vi "Set Snake Direction.vi"(8 "error in (no error)":errorcluster, 10 "Direction":T1, 11 "Snake in":refnum<class "Snake.lvclass">) -> (0 "error out":errorcluster, 3 "Snake out":refnum<class "Snake.lvclass">)   [LabVIEW 2018, in "Snake.lvclass"]
uses:
  Snake.lvclass
  Type Defs/Direction.ctl
  Snake.lvclass/Snake.ctl
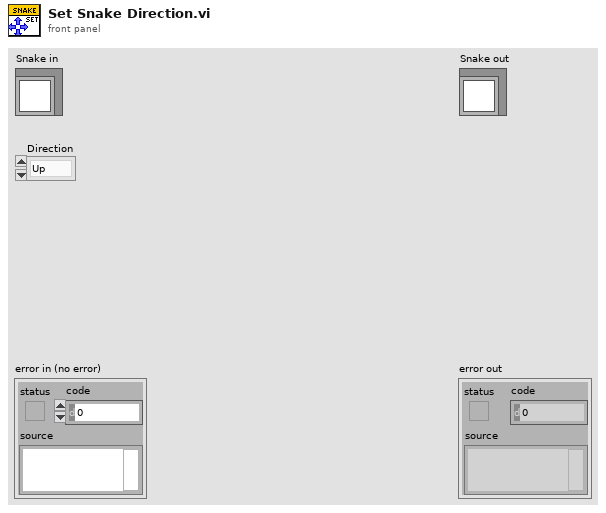
[diagram p1: front panel]
types:
  T1 = typedef "Direction.ctl" = enum16{"Up", "Down", "Left", "Right"}
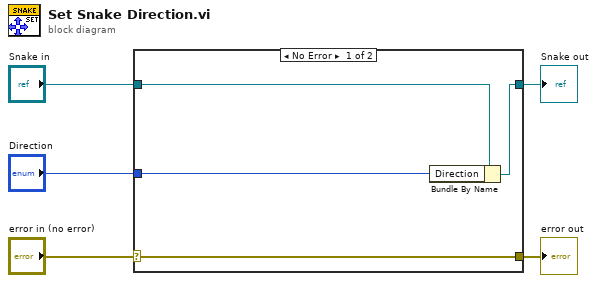
[diagram p0: block diagram]
diagram:
  n1 = case shown="No Error" "error in (no error)" {
    selector: "error in (no error)" -> [w9 w10]
    tunnel: [w9 w10] -> w4
    tunnel: [w7 w11] -> w2
    tunnel: "Snake in" -> [w8 w11]
    tunnel: "Direction" -> [w6 _]
    frame No Error {
      n2 = Bundle By Name(cluster=w8, "Direction"=w6) -> (w7:refnum<class "Snake.lvclass">)
    }
    frame Error {
    }
  }
  "error out" <- w4
  "Snake out" <- w2
